vi "RP100.TestLauncher.vi"() -> ()   [LabVIEW 2019, in "RP100.lvclass"]
uses:
  RP100.lvclass
  <vilib>/JKI/JKI SMO/SMO/SMO.lvclass
  <vilib>/JKI/JKI SMO/SMO/Typedefs/SMOState --Enum.ctl
  <userlib>/LevyLab/Levylab Instruments/SMOs/Instrument/Instrument.lvclass
  C:/Program Files (x86)/National Instruments/LabVIEW 2019/vi.lib/JKI/JKI SMO/SMO/SMO.lvclass
  C:/Program Files (x86)/National Instruments/LabVIEW 2019/user.lib/LevyLab/Levylab Instruments/SMOs/Instrument/Instrument.lvclass
  455319af-ff09-408a-88ef-82ea8c5cbc65.vi
  Typedefs/getAll.ctl
  86c5c1f9-8aa7-4fc6-95fb-80cd09b0b29c.vi
panel:
  out "measured I (A)":dbl format="%#_6p"
  out "measured I (A)":dbl format="%#_6p"
  out "measured V (V)":dbl format="%#_6p"
  out "measured V (V)":dbl format="%#_6p"
  out "Slew (V/s)":dbl format="%#_6p"
  out "Slew (V/s)":dbl format="%#_6p"
  out "Level (V)":dbl format="%#_6p"
  out "Level (V)":dbl format="%#_6p"
  out "Output State":string
  out "Output State":string
  out "SMO State":T1
  out "error out":errorcluster
  # "Razorbill Monitor"
  # "Channel 2"
  # "Channel 1"
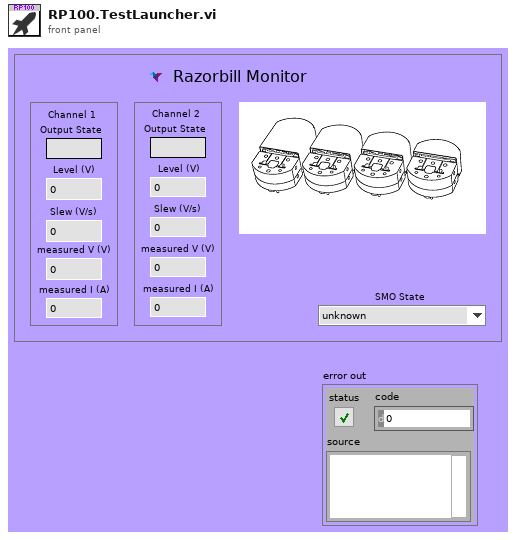
[diagram p1: front panel]
types:
  T1 = typedef "SMO.lvclass/SMOState --Enum.ctl" = enum16{"unknown", "Created", "Started", "Stopped"}
  T2 = typedef "SMO.lvclass/Public Events.ctl" = cluster{"Error":refnum<user-event>, "State":refnum<user-event>, "Reserve State":refnum<user-event>}
  T3 = typedef "Instrument.lvclass/PublicEvents--Cluster.ctl" = cluster{"MessageFromProcess":refnum<user-event>}
  T4 = cluster{"Event Registration Refnum":refnum<event-registration>}
  T5 = typedef "RP100.lvclass/getAll.ctl" = cluster{"Output State Ch1":string, "Output State Ch2":string, "Level (V) Ch1":dbl, "Level (V) Ch2":dbl, "Slew (V/s) Ch1":dbl, "Slew (V/s) Ch2":dbl, "measured V Ch1":dbl, "measured V Ch2":dbl, "measured I Ch1":dbl, "measured I Ch2":dbl}
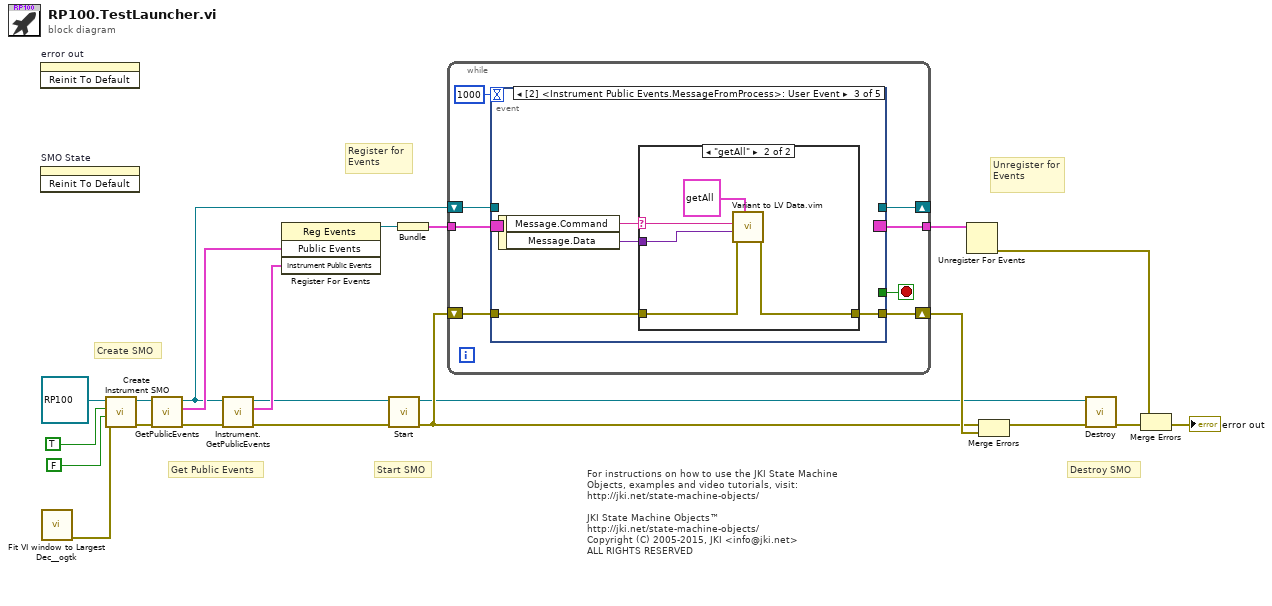
[diagram p0: block diagram]
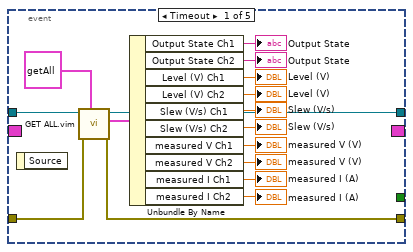
[diagram p2: hidden frame]
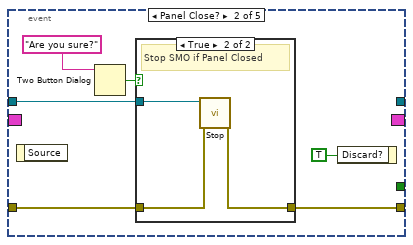
[diagram p3: hidden frame]
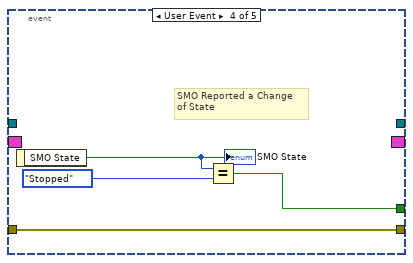
[diagram p6: hidden frame]
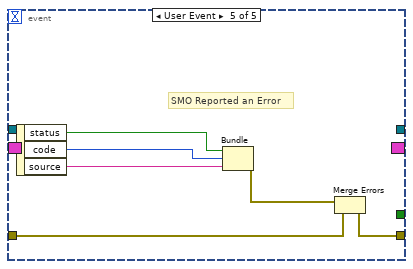
[diagram p7: hidden frame]
diagram:
  # "For instructions on how to use the JKI State Machine Objects, examples and video tutorials, visit:\nhttp://jki.net/state-machine-objects/\n\nJKI State Machine Objects™\nhttp://jki.net/state-machine-objects/\nCopyright (C) 2005-2015, JKI <info@jki.net>\nALL RIGHTS RESERVED"
  # "Get Public Events"
  # "Start SMO"
  # "Destroy SMO"
  # "Create SMO"
  # "Unregister for Events"
  # "Register for Events"
  n1 = invoke on="error out" class="Clust (strict)" method="Reinit To Default"() -> ()  [unwired: 3 in, 3 out]
  n2 = invoke on="SMO State" class="Enum (strict)" method="Reinit To Default"() -> ()  [unwired: 3 in, 3 out]
  n3 = call <userlib>:"Fit VI window to Largest Dec__ogtk.vi"() -> ("error out"=w6:errorcluster)  [unwired: 6 in, 1 out]
  n4 = call-dynamic "Create Instrument SMO.vi"("error in (no error)"=w6, "Debug Mode? [F]"=FALSE, "Configuration Window? [T]"=TRUE, "Instrument in"=refnum<class "RP100.lvclass"> refnum ("SMO.Template.lvclass")) -> ("error out"=w9:errorcluster, "Instrument out"=w10:refnum<class "RP100.lvclass">)  [unwired: 6 in]
  n5 = call <vilib>:"GetPublicEvents.vi"("error in (no error)"=w9, "SMO"=w10) -> ("error out"=w4:errorcluster, "Public Events"=w13:T2, "SMO out"=w5:refnum<class "RP100.lvclass">)  [unwired: 7 in]
  n6 = call <userlib>:"Instrument.GetPublicEvents.vi"("error in (no error)"=w4, "Instrument"=w5) -> ("error out"=w1:errorcluster, "Instrument Public Events"=w3:T3, "Instrument out"=w2:refnum<class "RP100.lvclass">)  [unwired: 7 in]
  n7 = register-events(w13, w3) -> (reference out=w12:refnum<event-registration>)  [unwired: 2 in, 1 out]
  n8 = call <vilib>:"Start.vi"("error in (no error)"=w1, "SMO"=w2) -> ("error out"=w16:errorcluster, "SMO out"=w14:refnum<class "RP100.lvclass">)  [unwired: 8 in]
  n9 = Bundle("Event Registration Refnum"=w12) -> (w21:T4)  [unwired: 1 in]
  n10 = while {
    shift-right: [w29] -> w20
    shift-left: w16 -> [w28]
    tunnel: w21 -> [w27]
    tunnel: [w26] -> w22
    shift-right: [w23] -> _
    shift-left: w5 -> [w25]
    stop <- w30 stop-if-true
    n11 = event shown="[2] <Instrument Public Events.MessageFromProcess>: User Event" {
      selector: w27 -> [_ _ _ _ _]
      dyn-events: [_ _ _ _ _] -> w26
      timeout: 1000 -> [_ _ _ _ _]
      tunnel: [_ _ _ w67 _] -> w30
      tunnel: w25 -> [w46 w52 _ _ _]
      tunnel: [w33 w51 w57 w70 w75] -> w29
      tunnel: w28 -> [w32 w50 w58 w70 w71]
      tunnel: [w31 _ _ _ _] -> w23
      event Timeout {
        n12 = event-data() -> ()  [unwired: 1 in, 1 out]
        n13 = call "GET ALL.vim"("type"=T5 {"Output State Ch1"="", "Output State Ch2"="", "Level (V) Ch1"=0.0, "Level (V) Ch2"=0.0, "Slew (V/s) Ch1"=0.0, "Slew (V/s) Ch2"=0.0, "measured V Ch1"=0.0, "measured V Ch2"=0.0, "measured I Ch1"=0.0, "measured I Ch2"=0.0} ("Cluster"), "error in (no error)"=w32, "Instrument in"=w46) -> ("error out"=w33:errorcluster, "getAll"=w44:T5, "Instrument out"=w31:refnum<class "RP100.lvclass">)  [unwired: 6 in]
        n14 = Unbundle By Name(w44) -> ("Output State Ch1"=→"Output State":string, "Output State Ch2"=→"Output State":string, "Level (V) Ch1"=→"Level (V)":dbl, "Level (V) Ch2"=→"Level (V)":dbl, "Slew (V/s) Ch1"=→"Slew (V/s)":dbl, "Slew (V/s) Ch2"=→"Slew (V/s)":dbl, "measured V Ch1"=→"measured V (V)":dbl, "measured V Ch2"=→"measured V (V)":dbl, "measured I Ch1"=→"measured I (A)":dbl, "measured I Ch2"=→"measured I (A)":dbl)
      }
      event Panel Close? {
        n15 = event-data() -> ()  [unwired: 1 in, 1 out]
        n16 = Two Button Dialog(message="Are you sure?") -> (T button?=w48:bool)  [unwired: 2 in]
        n17 = case shown="True" w48 {
          tunnel: w52 -> [_ w56]
          tunnel: [w53 w55] -> w51
          tunnel: w50 -> [w53 w54]
          frame False {
          }
          frame True {
            # "Stop SMO if Panel Closed"
            n18 = call <vilib>:"Stop.vi"("error in (no error)"=w54, "SMO"=w56) -> ("error out"=w55:errorcluster)  [unwired: 8 in, 1 out]
          }
        }
        n19 = event-data("Discard?"=TRUE ("OK")) -> ()  [unwired: 1 in, 1 out]
      }
      event User Event {
        n20 = event-data() -> ("Message.Command"=w60:string, "Message.Data"=w59:variant)  [unwired: 1 in]
        n21 = case shown="\"getAll\"" w60 {
          selector: w60 -> [_ w65]
          tunnel: w59 -> [_ w64]
          tunnel: w58 -> [w61 w62]
          tunnel: [w61 w63] -> w57
          frame Default {
          }
          frame "getAll" {
            n22 = call "Variant to LV Data.vim"("type"=T5 {"Output State Ch1"="", "Output State Ch2"="", "Level (V) Ch1"=0.0, "Level (V) Ch2"=0.0, "Slew (V/s) Ch1"=0.0, "Slew (V/s) Ch2"=0.0, "measured V Ch1"=0.0, "measured V Ch2"=0.0, "measured I Ch1"=0.0, "measured I Ch2"=0.0} ("Cluster"), "error in (no error)"=w62, "JSON Data in"=w64, "Command"=w65) -> ("error out"=w63:errorcluster)  [unwired: 4 in, 3 out]
          }
        }
      }
      event User Event {
        # "SMO Reported a Change\nof State"
        n23 = event-data() -> ("SMO State"=w69:T1)  [unwired: 1 in]
        "SMO State" <- w69
        n24 = Equal?(x=w69, y=SMOState_--Enum."Stopped") -> (x = y?=w67:bool)
      }
      event User Event {
        # "SMO Reported an Error"
        n25 = event-data() -> ("status"=w74:bool, "code"=w73:i32, "source"=w76:string)  [unwired: 1 in]
        n26 = Bundle("status"=w74, "code"=w73, "source"=w76) -> (w72:errorcluster)  [unwired: 1 in]
        n27 = Merge Errors(w72, w71) -> (w75:errorcluster)
      }
    }
  }
  n28 = Unregister For Events(event registration refnum=w22) -> (error out=w19:errorcluster)  [unwired: 1 in]
  n29 = Merge Errors(w16, w20) -> (w15:errorcluster)
  n30 = call <vilib>:"Destroy.vi"("error in (no error)"=w15, "SMO"=w14) -> ("error out"=w17:errorcluster)  [unwired: 9 in]
  n31 = Merge Errors(w19, w17) -> (→"error out":errorcluster)
